vi "Simple_Initialize.vi"(7 "PwrSns Model RegEx":string, 8 "error in (no error)":errorcluster, 9 "Reset (True)":bool=TRUE, 10 "ID Query (True)":bool=TRUE, 11 "VISA resource name":refnum<visa-resource-name>) -> (0 "error out":errorcluster, 3 "VISA resource name out":refnum<visa-resource-name>)   [LabVIEW 2025, in "Interface Functions.lvlib"]
doc: "Establishes communication with the instrument and optionally performs an instrument identification query and/or an instrument reset. It also places the instrument in a default state needed for other instrument driver operations. Therefore, call this VI before calling other instrument driver VIs for this instrument. Generally, you need to call the Initialize VI only once at the beginning of an application."
uses:
  Interface Functions.lvlib
  <vilib>/regexp/Match Regular Expression.xnode
  <instrlib>/Agilent U2000 Series/Agilent U2000 Series.lvlib
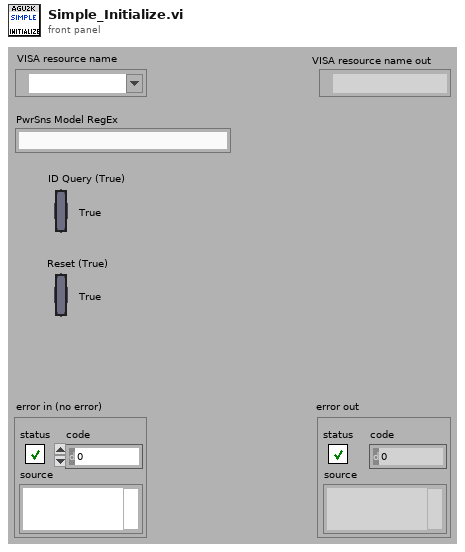
[diagram p1: front panel]
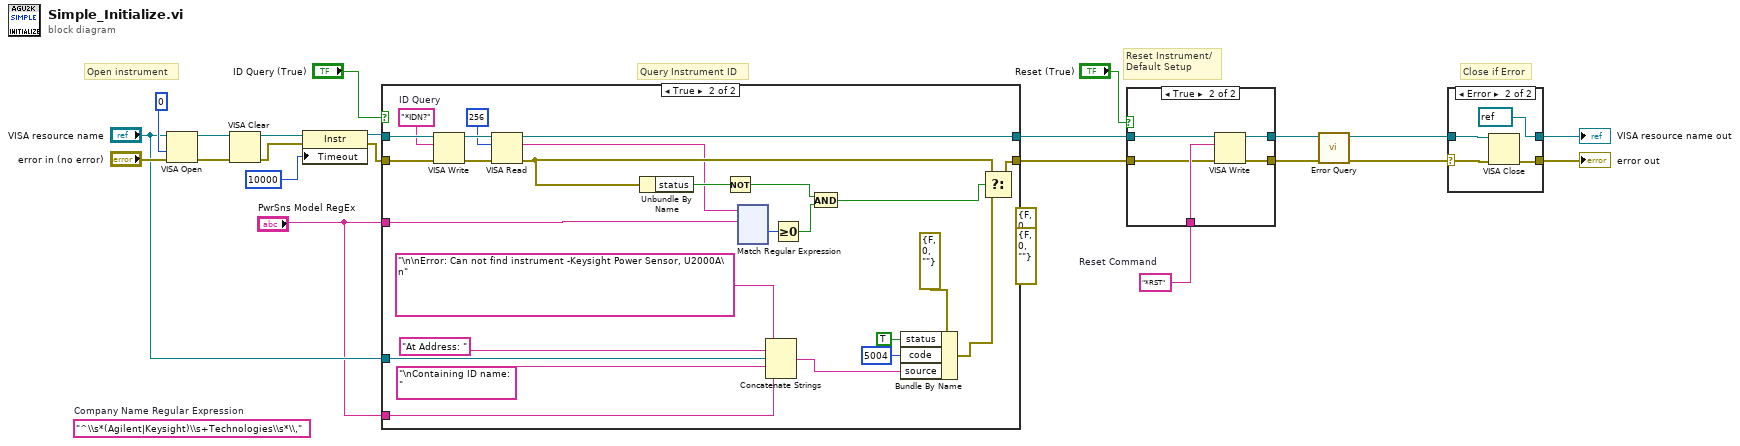
[diagram p0: block diagram]
diagram:
  (unwired) "^\\s*(Agilent|Keysight)\\s+Technologies\\s*\\,"  # Company Name Regular Expression
  w7 = "*RST"  # Reset Command
  # "Close if Error"
  # "Query Instrument ID"
  # "Reset Instrument/\nDefault Setup"
  # "Open instrument"
  n1 = VISA Open(access mode=u32 0, error in (no error)="error in (no error)", VISA resource name="VISA resource name") -> (VISA resource name=w18:refnum<visa-resource-name>, error out=w17:errorcluster)  [unwired: 2 out]
  n2 = VISA Clear(VISA resource name=w18, error in (no error)=w17) -> (VISA resource name out=w14:refnum<visa-resource-name>, error out=w13:errorcluster)
  n3 = property class="Instr"(reference=w14, error in=w13, "Timeout"=u32 10000 ("General Settings:Timeout Value")) -> (reference out=w11:refnum<visa-resource-name>, error out=w10:errorcluster)
  n4 = case shown="True" "ID Query (True)" {
    tunnel: [w23 w50] -> w8
    tunnel: [w24 w47] -> w9
    tunnel: w11 -> [w24 w48]
    tunnel: w10 -> [w23 w49]
    tunnel: "PwrSns Model RegEx" -> [_ w36]
    tunnel: "VISA resource name" -> [_ w28]
    tunnel: "PwrSns Model RegEx" -> [_ w26]
    frame False {
    }
    frame True {
      (unwired) errorcluster {"status"=FALSE, "code"=0, "source"=""} ("error out")
      (unwired) errorcluster {"status"=FALSE, "code"=0, "source"=""} ("error out")
      w43 = "*IDN?"  # ID Query
      n5 = VISA Write(VISA resource name=w48, write buffer=w43, error in (no error)=w49) -> (VISA resource name out=w46:refnum<visa-resource-name>, error out=w45:errorcluster)  [unwired: 1 out]
      n6 = VISA Read(VISA resource name=w46, byte count=u32 256, error in (no error)=w45) -> (VISA resource name out=w47:refnum<visa-resource-name>, read buffer=w37:string, error out=w42:errorcluster)  [unwired: 1 out]
      n7 = Unbundle By Name(w42) -> ("status"=w41:bool)
      n8 = Not(x=w41) -> (.not. x?=w35:bool)
      n9 = xnode "Match Regular Expression"("input string"=w37, "regular expression"=w36) -> ("offset past match"=w38:i32)  [unwired: 4 in, 4 out]
      n10 = Concatenate Strings("\n\nError: Can not find instrument -Keysight Power Sensor, U2000A\n", "At Address: ", w28, "\nContaining ID name: ", w26) -> (w25:string)
      n11 = Greater Or Equal To 0?(x=w38) -> (x >= 0?=w40:bool)
      n12 = And(x=w35, y=w40) -> (x .and. y?=w39:bool)
      n13 = Bundle By Name(cluster=errorcluster {"status"=FALSE, "code"=0, "source"=""} ("error out"), "status"=TRUE, "code"=5004, "source"=w25) -> (w33:errorcluster)
      n14 = Select(t=w42, s=w39, f=w33) -> (s? t:f=w50:errorcluster)
    }
  }
  n15 = case shown="True" "Reset (True)" {
    tunnel: w8 -> [w168 w171]
    tunnel: [w168 w173] -> w5
    tunnel: w9 -> [w169 w170]
    tunnel: [w169 w174] -> w6
    tunnel: w7 -> [_ w172]
    frame False {
    }
    frame True {
      n16 = VISA Write(VISA resource name=w170, write buffer=w172, error in (no error)=w171) -> (VISA resource name out=w174:refnum<visa-resource-name>, error out=w173:errorcluster)  [unwired: 1 out]
    }
  }
  n17 = call <instrlib>:"Error Query.vi"("error in (no error)"=w5, "VISA resource name"=w6) -> ("error out"=w3:errorcluster, "VISA resource name out"=w4:refnum<visa-resource-name>)  [unwired: 8 out]
  n18 = case shown="Error" w3 {
    selector: w3 -> [w175 w178]
    tunnel: w4 -> [w176 w179]
    tunnel: [w176 refnum<visa-resource-name> refnum ("VISA resource name out")] -> w16
    tunnel: [w175 w177] -> w15
    frame No Error {
    }
    frame Error {
      n19 = VISA Close(VISA resource name=w179, error in (no error)=w178) -> (error out=w177:errorcluster)
    }
  }
  "VISA resource name out" <- w16
  "error out" <- w15
